vi "From String.vi"(6 "CConfig Encoding [Automatic]":refnum<class "CConfig Encoding.lvclass">=refnum, 8 "error in (no error)":errorcluster, 10 "String":string) -> (0 "error out":errorcluster, 2 "Used encoding":refnum<class "CConfig Encoding.lvclass">, 3 "Section Object out":refnum<class "CConfig Object.lvclass">)   [LabVIEW 2013, in "CConfig Object.lvclass"]
doc: "Copyright 2018, Carya Automatisering, Wiebe Walstra."
uses:
  CConfig Object.lvclass
  CConfig Encoding/CConfig Encoding.lvclass
  CConfig Encoding/CConfig Automatic Encoding/CConfig Automatic Encoding.lvclass
  Data.ctl
  Loop Query/Loop Query.lvclass
  Loop Query/Match Query/Match Query.lvclass
  Insert Query/Insert Query.lvclass
  Set Query/Set Query.lvclass
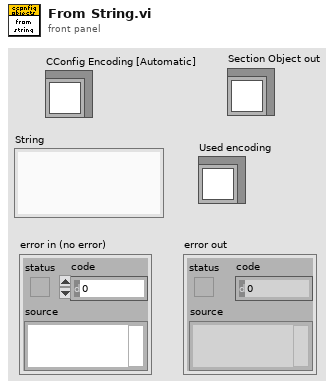
[diagram p1: front panel]
types:
  T1 = typedef "CConfig Object.lvclass/Data.ctl" = enum16{"pre", "name", "middle", "value", "post", "newline", "persistant", "tagged", "type"}
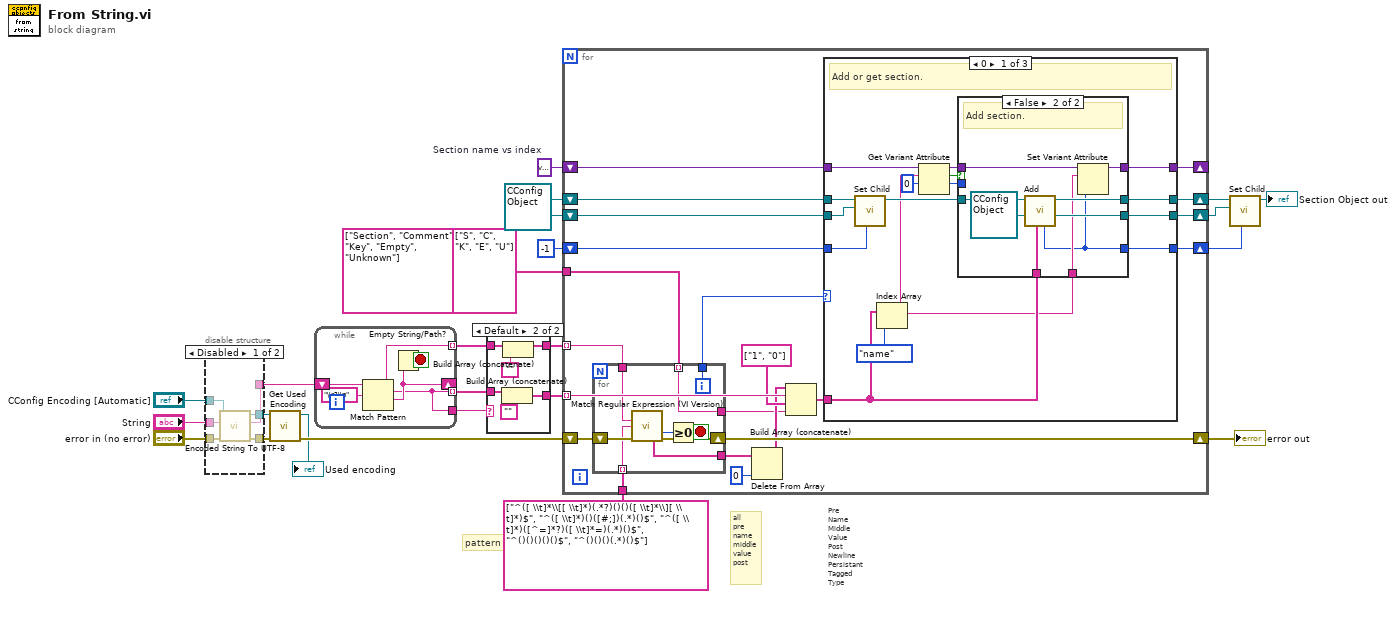
[diagram p0: block diagram]
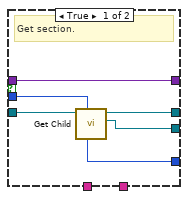
[diagram p3: hidden frame]
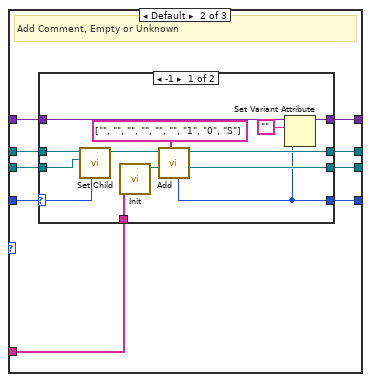
[diagram p4: hidden frame]
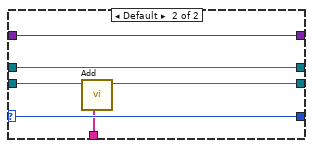
[diagram p5: hidden frame]
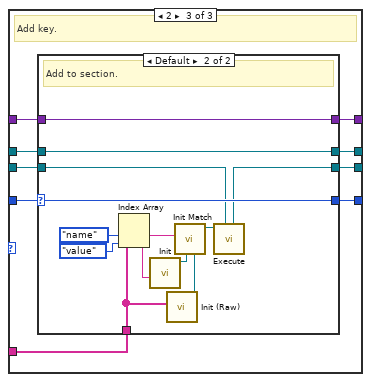
[diagram p6: hidden frame]
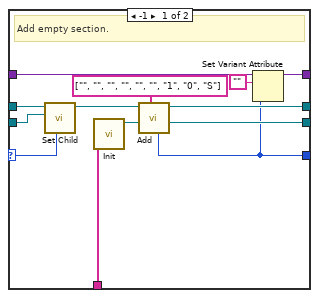
[diagram p7: hidden frame]
diagram:
  w10 = variant  # Section name vs index
  (unwired) string[] ["Section", "Comment", "Key", "Empty", "Unknown"] ("Array 2")
  w11 = refnum<class "CConfig Object.lvclass"> refnum
  # "pattern for type"
  # "Pre\nName\nMiddle\nValue\nPost\nNewline\nPersistant\nTagged\nType"
  # "all\npre\nname\nmiddle\nvalue\npost"
  n1 = disable-structure shown="Disabled" {
    disable-tunnel: "error in (no error)" -> [w29 w30]
    disable-tunnel: "String" -> [w28 w31]
    disable-tunnel: [w27 w31] -> w7
    disable-tunnel: "CConfig Encoding [Automatic]" -> [w26 _]
    disable-tunnel: [w25 _] -> w4
    disable-tunnel: [w24 w30] -> w3
    frame Disabled {
      n2 = call-dynamic "Encoded String To UTF-8.vi"("error in (no error)"=w29, "Encoded string"=w28, "Encoding in"=w26) -> ("error out"=w24:errorcluster, "UTF-8 string"=w27:string, "Encoding out"=w25:refnum<class "CConfig Encoding.lvclass">)  [unwired: 6 in]
    }
    frame Enabled {
    }
  }
  n3 = call-dynamic "Get Used Encoding.vi"("error in (no error)"=w3, "CConfig Encoding in"=w4) -> ("error out"=w2:errorcluster, "CConfig Encoding out"=→"Used encoding":refnum<class "CConfig Encoding.lvclass">)  [unwired: 8 in]
  n4 = while {
    shift-right: [w34] -> _
    shift-left: w7 -> [w37]
    tunnel: [w33] -> w21 mode=indexing
    tunnel: [w32] -> w6
    tunnel: [w32] -> w20 mode=indexing
    stop <- w35 stop-if-true
    n5 = Match Pattern(string=w37, regular expression="\\r?\\n") -> (before substring=w33:string, match substring=w32:string, after substring=w34:string)  [unwired: 1 in, 1 out]
    n6 = Empty String/Path?(string/path=w34) -> (empty?=w35:bool)
  }
  n7 = case shown="Default" w6 {
    tunnel: w21 -> [w39 w45]
    tunnel: [w39 w44] -> w19
    tunnel: w20 -> [w38 w42]
    tunnel: [w38 w41] -> w18
    frame "" {
    }
    frame Default {
      n8 = Build Array (concatenate)(w42, "") -> (w41:string[])
      n9 = Build Array (concatenate)(w45, "") -> (w44:string[])
    }
  }
  n10 = for {
    tunnel: string[] ["^([ \\t]*\\[[ \\t]*)(.*?)()()([ \\t]*\\][ \\t]*)$", "^([ \\t]*)()([#;])(.*)()$", "^([ \\t]*)([^=]*?)([ \\t]*=)(.*)()$", "^()()()()()$", "^()()()(.*)()$"] -> [w64]
    tunnel: string[] ["S", "C", "K", "E", "U"] ("Array") -> [w63]
    tunnel: w19 -> [w62] mode=indexing
    tunnel: w18 -> [w61] mode=indexing
    shift-right: [w52] -> w15
    shift-left: w11 -> [w53]
    shift-right: [w51] -> w12
    shift-left: -1 ("Index") -> [w50]
    shift-right: [w65] -> w23
    shift-left: w2 -> [w66]
    shift-right: [w49] -> w13
    shift-left: w11 -> [w48]
    shift-right: [w46] -> _
    shift-left: w10 -> [w47]
    n11 = for {
      shift-right: [w164] -> w65
      shift-left: w66 -> [w165]
      tunnel: w64 -> [w163] mode=indexing
      tunnel: [w159] -> w58
      tunnel: w62 -> [w162]
      tunnel: w63 -> [w158] mode=indexing
      tunnel: [w158] -> w56
      tunnel: [w157] -> w54
      i -> [w157]
      stop <- w160 stop-if-true
      n12 = call "Match Regular Expression (VI Version).vi"("input string"=w162, "regular expression"=w163, "error in"=w165) -> ("offset past match"=w161:i32, "Capturing goups"=w159:string[], "error out"=w164:errorcluster)  [unwired: 6 in, 4 out]
      n13 = Greater Or Equal To 0?(x=w161) -> (x >= 0?=w160:bool)
    }
    n14 = Delete From Array(array=w58, index=0) -> (array with subset deleted=w59:string[])  [unwired: 1 in, 1 out]
    n15 = Build Array (concatenate)(w59, w61, string[] ["1", "0"], w56) -> (w55:string[])
    n16 = case shown="0" w54 {
      tunnel: w55 -> [w81 w104 w131]
      tunnel: w53 -> [w78 w103 w130]
      tunnel: [w75 w101 w128] -> w52
      tunnel: [w80 w102 w129] -> w51
      tunnel: w50 -> [w76 w100 w127]
      tunnel: [w74 w98 w125] -> w49
      tunnel: w48 -> [w77 w99 w126]
      tunnel: w47 -> [w73 w97 w124]
      tunnel: [w67 w96 w123] -> w46
      frame 0 {
        # "Add or get section."
        n17 = call-dynamic "Set Child.vi"("Index in"=w76, "Child"=w77, "Composite Object in"=w78) -> ("Composite Object out"=w79:refnum<class "CConfig Object.lvclass">)  [unwired: 7 in, 1 out]
        n18 = Index Array(array=w81, index=Data."name" ("Data [name[")) -> (element=w72:string)
        n19 = Get Variant Attribute(Variant=w73, name=w72, default value (empty Variant)=0) -> (duplicate Variant=w68:variant, found=w71:bool, value=w69:i32)  [unwired: 1 in, 1 out]
        n20 = case shown="False" w71 {
          tunnel: [w86 w94] -> w75
          tunnel: w79 -> [w87 w95]
          tunnel: w81 -> [_ w92]
          tunnel: [w84 w88] -> w80
          tunnel: w72 -> [_ w89]
          tunnel: [w85 w93] -> w74
          tunnel: w69 -> [w84 _]
          tunnel: w68 -> [w83 w91]
          tunnel: [w83 w90] -> w67
          frame True {
            # "Get section."
            n21 = call-dynamic "Get Child.vi"("Index in"=w84, "Composite Object in"=w87) -> ("Child"=w85:refnum<class "CConfig Object.lvclass">, "Composite Object out"=w86:refnum<class "CConfig Object.lvclass">)  [unwired: 7 in, 1 out]
          }
          frame False {
            w93 = refnum<class "CConfig Object.lvclass"> refnum ("Composite Object.lvclass")
            # "Add section."
            n22 = call-dynamic "Add.vi"("Data"=w92, "Child"=w93, "Composite Object in"=w95) -> ("Composite Object out"=w94:refnum<class "CConfig Object.lvclass">, "Index"=w88:i32)  [unwired: 6 in, 1 out]
            n23 = Set Variant Attribute(Variant=w91, name=w89, value=w88) -> (Variant out=w90:variant)  [unwired: 1 in, 2 out]
          }
        }
      }
      frame Default {
        # "Add Comment, Empty or Unknown"
        n24 = case shown="-1" w100 {
          selector: w100 -> [w110 w122]
          tunnel: w104 -> [w116 w118]
          tunnel: w103 -> [w112 w119]
          tunnel: [w106 w122] -> w102
          tunnel: [w115 w119] -> w101
          tunnel: w97 -> [w108 w117]
          tunnel: w99 -> [w111 w121]
          tunnel: [w114 w120] -> w98
          tunnel: [w107 w117] -> w96
          frame -1 {
            n25 = call-dynamic "Set Child.vi"("Index in"=w110, "Child"=w111, "Composite Object in"=w112) -> ("Composite Object out"=w113:refnum<class "CConfig Object.lvclass">)  [unwired: 7 in, 1 out]
            n26 = call "Init.vi"("Data"=w116) -> ("Composite Object out"=w114:refnum<class "CConfig Object.lvclass">)  [unwired: 9 in, 1 out]
            n27 = call-dynamic "Add.vi"("Data"=string[] ["", "", "", "", "", "", "1", "0", "S"], "Child"=w114, "Composite Object in"=w113) -> ("Composite Object out"=w115:refnum<class "CConfig Object.lvclass">, "Index"=w106:i32)  [unwired: 6 in, 1 out]
            n28 = Set Variant Attribute(Variant=w108, name="", value=w106) -> (Variant out=w107:variant)  [unwired: 1 in, 2 out]
          }
          frame Default {
            n29 = call-dynamic "Add.vi"("Data"=w118, "Composite Object in"=w121) -> ("Composite Object out"=w120:refnum<class "CConfig Object.lvclass">)  [unwired: 7 in, 2 out]
          }
        }
      }
      frame 2 {
        # "Add key."
        n30 = case shown="Default" w127 {
          selector: w127 -> [w137 w156]
          tunnel: w131 -> [w143 w152]
          tunnel: w130 -> [w140 w144]
          tunnel: [w133 w156] -> w129
          tunnel: [w142 w144] -> w128
          tunnel: [w134 w155] -> w123
          tunnel: w124 -> [w135 w155]
          tunnel: w126 -> [w138 w146]
          tunnel: [w141 w145] -> w125
          frame -1 {
            # "Add empty section."
            n31 = call-dynamic "Set Child.vi"("Index in"=w137, "Child"=w138, "Composite Object in"=w140) -> ("Composite Object out"=w139:refnum<class "CConfig Object.lvclass">)  [unwired: 7 in, 1 out]
            n32 = call "Init.vi"("Data"=w143) -> ("Composite Object out"=w141:refnum<class "CConfig Object.lvclass">)  [unwired: 9 in, 1 out]
            n33 = call-dynamic "Add.vi"("Data"=string[] ["", "", "", "", "", "", "1", "0", "S"], "Child"=w141, "Composite Object in"=w139) -> ("Composite Object out"=w142:refnum<class "CConfig Object.lvclass">, "Index"=w133:i32)  [unwired: 6 in, 1 out]
            n34 = Set Variant Attribute(Variant=w135, name="", value=w133) -> (Variant out=w134:variant)  [unwired: 1 in, 2 out]
          }
          frame Default {
            # "Add to section."
            n35 = Index Array(array=w152, index #1=Data."name" ("Data [name["), index #2=Data."value" ("Data [name[")) -> (element #1=w151:string, element #2=w150:string)
            n36 = call "Init.vi"("Value"=w150) -> ("Set Query out"=w149:refnum<class "Set Query.lvclass">)  [unwired: 9 in, 1 out]
            n37 = call "Init (Raw).vi"("Data"=w152) -> ("Find First Query out"=w153:refnum<class "Insert Query.lvclass">)  [unwired: 9 in, 1 out]
            n38 = call "Init Match.vi"("Not found"=w153, "Found"=w149, "Data"=w151) -> ("Find First Query out"=w154:refnum<class "Loop Query.lvclass">)  [unwired: 7 in, 1 out]
            n39 = call-dynamic "Execute.vi"("Composite Object"=w146, "Config Query in"=w154) -> ("Composite Object"=w145:refnum<class "CConfig Object.lvclass">)  [unwired: 4 in, 5 out]
          }
        }
      }
    }
  }
  "error out" <- w23
  n40 = call-dynamic "Set Child.vi"("Index in"=w12, "Child"=w13, "Composite Object in"=w15) -> ("Composite Object out"=→"Section Object out":refnum<class "CConfig Object.lvclass">)  [unwired: 7 in, 1 out]
